vi "XMLExtractSheetData.vi"(8 "error in (no error)":errorcluster, 11 "SheetsXML":string[](array[string])=["<table:table table:name=\"Sheet1\" table:style-name=\"ta1\"><table:table-column table:style-name=\"co1\" table:number-columns-repeated=\"8\" table:default-cell-style-name=\"Default\"/><table:table-row table:style-name=\"ro1\" table:number-rows-repeated=\"3\"><table:table-cell table:number-columns-repeated=\"8\"/></table:table-row><table:table-row table:style-name=\"ro1\"><table:table-cell/><table:table-cell office:value-type=\"string\" calcext:value-type=\"string\"><text:p>b1</text:p></table:table-cell><table:table-cell office:value-type=\"string\" calcext:value-type=\"string\"><text:p>c1</text:p></table:table-cell><table:table-cell table:number-columns-repeated=\"5\"/></table:table-row><table:table-row table:style-name=\"ro1\"><table:table-cell/><table:table-cell office:value-type=\"string\" calcext:value-type=\"string\"><text:p>b2</text:p></table:table-cell><table:table-cell office:value-type=\"string\" calcext:value-type=\"string\"><text:p>c2</text:p></table:table-cell><table:table-cell table:number-columns-repeated=\"5\"/></table:table-row><table:table-row table:style-name=\"ro1\"><table:table-cell/><table:table-cell office:value-type=\"string\" calcext:value-type=\"string\"><text:p>b3</text:p></table:table-cell><table:table-cell office:value-type=\"string\" calcext:value-type=\"string\"><text:p>c3</text:p></table:table-cell><table:table-cell table:number-columns-repeated=\"5\"/></table:table-row><table:table-row table:style-name=\"ro1\"><table:table-cell/><table:table-cell office:value-type=\"string\" calcext:value-type=\"string\"><text:p>b4</text:p></table:table-cell><table:table-cell office:value-type=\"string\" calcext:value-type=\"string\"><text:p>c4</text:p></table:table-cell><table:table-cell table:number-columns-repeated=\"5\"/></table:table-row><table:table-row table:style-name=\"ro1\"><table:table-cell/><table:table-cell office:value-type=\"string\" calcext:value-type=\"string\"><text:p>b5</text:p></table:table-cell><table:table-cell office:value-type=\"string\" calcext:value-type=\"string\"><text:p>c5</text:p></table:table-cell><table:table-cell table:number-columns-repeated=\"5\"/></table:table-row><table:table-row table:style-name=\"ro1\"><table:table-cell/><table:table-cell office:value-type=\"string\" calcext:value-type=\"string\"><text:p>b6</text:p></table:table-cell><table:table-cell office:value-type=\"string\" calcext:value-type=\"string\"><text:p>c6</text:p></table:table-cell><table:table-cell table:number-columns-repeated=\"5\"/></table:table-row><table:table-row table:style-name=\"ro1\"><table:table-cell/><table:table-cell office:value-type=\"string\" calcext:value-type=\"string\"><text:p>b7</text:p></table:table-cell><table:table-cell office:value-type=\"string\" calcext:value-type=\"string\"><text:p>c7</text:p></table:table-cell><table:table-cell table:number-columns-repeated=\"5\"/></table:table-row><table:table-row table:style-name=\"ro1\"><table:table-cell/><table:table-cell office:value-type=\"string\" calcext:value-type=\"string\"><text:p>b8</text:p></table:table-cell><table:table-cell office:value-type=\"string\" calcext:value-type=\"string\"><text:p>c8</text:p></table:table-cell><table:table-cell table:number-columns-repeated=\"5\"/></table:table-row><table:table-row table:style-name=\"ro1\" table:number-rows-repeated=\"2\"><table:table-cell table:number-columns-repeated=\"8\"/></table:table-row><table:table-row table:style-name=\"ro1\"><table:table-cell table:number-columns-repeated=\"3\"/><table:table-cell office:value-type=\"string\" calcext:value-type=\"string\"><text:p>d1</text:p></table:table-cell><table:table-cell office:value-type=\"string\" calcext:value-type=\"string\"><text:p>e1</text:p></table:table-cell><table:table-cell table:number-columns-repeated=\"3\"/></table:table-row><table:table-row table:style-name=\"ro1\"><table:table-cell table:number-columns-repeated=\"3\"/><table:table-cell office:value-type=\"string\" calcext:value-type=\"string\"><text:p>d2</text:p></table:table-cell><table:table-cell office:value-type=\"string\" calcext:value-type=\"string\"><text:p>e2</text:p></table:table-cell><table:table-cell table:number-columns-repeated=\"3\"/></table:table-row><table:table-row table:style-name=\"ro1\"><table:table-cell table:number-columns-repeated=\"3\"/><table:table-cell office:value-type=\"string\" calcext:value-type=\"string\"><text:p>d3</text:p></table:table-cell><table:table-cell office:value-type=\"string\" calcext:value-type=\"string\"><text:p>e3</text:p></table:table-cell><table:table-cell table:number-columns-repeated=\"3\"/></table:table-row><table:table-row table:style-name=\"ro1\"><table:table-cell table:number-columns-repeated=\"3\"/><table:table-cell office:value-type=\"string\" calcext:value-type=\"string\"><text:p>d4</text:p></table:table-cell><table:table-cell office:value-type=\"string\" calcext:value-type=\"string\"><text:p>e4</text:p></table:table-cell><table:table-cell table:number-columns-repeated=\"3\"/></table:table-row><table:table-row table:style-name=\"ro1\"><table:table-cell table:number-columns-repeated=\"3\"/><table:table-cell office:value-type=\"string\" calcext:value-type=\"string\"><text:p>d5</text:p></table:table-cell><table:table-cell office:value-type=\"string\" calcext:value-type=\"string\"><text:p>e5</text:p></table:table-cell><table:table-cell table:number-columns-repeated=\"3\"/></table:table-row><table:table-row table:style-name=\"ro1\" table:number-rows-repeated=\"14\"><table:table-cell table:number-columns-repeated=\"8\"/></table:table-row><table:table-row table:style-name=\"ro1\"><table:table-cell table:number-columns-repeated=\"5\"/><table:table-cell office:value-type=\"string\" calcext:value-type=\"string\"><text:p>f1</text:p></table:table-cell><table:table-cell/><table:table-cell office:value-type=\"string\" calcext:value-type=\"string\"><text:p>h1</text:p></table:table-cell></table:table-row><table:table-row table:style-name=\"ro1\"><table:table-cell table:number-columns-repeated=\"5\"/><table:table-cell office:value-type=\"string\" calcext:value-type=\"string\"><text:p>f2</text:p></table:table-cell><table:table-cell/><table:table-cell office:value-type=\"string\" calcext:value-type=\"string\"><text:p>h2</text:p></table:table-cell></table:table-row><table:table-row table:style-name=\"ro1\"><table:table-cell table:number-columns-repeated=\"5\"/><table:table-cell office:value-type=\"string\" calcext:value-type=\"string\"><text:p>f3</text:p></table:table-cell><table:table-cell/><table:table-cell office:value-type=\"string\" calcext:value-type=\"string\"><text:p>h3</text:p></table:table-cell></table:table-row><table:table-row table:style-name=\"ro1\"><table:table-cell table:number-columns-repeated=\"5\"/><table:table-cell office:value-type=\"string\" calcext:value-type=\"string\"><text:p>f4</text:p></table:table-cell><table:table-cell/><table:table-cell office:value-type=\"string\" calcext:value-type=\"string\"><text:p>h4</text:p></table:table-cell></table:table-row><table:table-row table:style-name=\"ro1\"><table:table-cell table:number-columns-repeated=\"5\"/><table:table-cell office:value-type=\"string\" calcext:value-type=\"string\"><text:p>f5</text:p></table:table-cell><table:table-cell/><table:table-cell office:value-type=\"string\" calcext:value-type=\"string\"><text:p>h5</text:p></table:table-cell></table:table-row><table:table-row table:style-name=\"ro1\"><table:table-cell table:number-columns-repeated=\"5\"/><table:table-cell office:value-type=\"string\" calcext:value-type=\"string\"><text:p>f6</text:p></table:table-cell><table:table-cell/><table:table-cell office:value-type=\"string\" calcext:value-type=\"string\"><text:p>h6</text:p></table:table-cell></table:table-row><table:table-row table:style-name=\"ro1\"><table:table-cell table:number-columns-repeated=\"5\"/><table:table-cell office:value-type=\"string\" calcext:value-type=\"string\"><text:p>f7</text:p></table:table-cell><table:table-cell/><table:table-cell office:value-type=\"string\" calcext:value-type=\"string\"><text:p>h7</text:p></table:table-cell></table:table-row></table:table>"]) -> (0 "error out":errorcluster, 2 "SpreadsheetData":T1[](array[typedef]), 3 "Table HeaderInfo":string[](array[string]))   [LabVIEW 2014]
uses:
  Spreadsheets.ctl
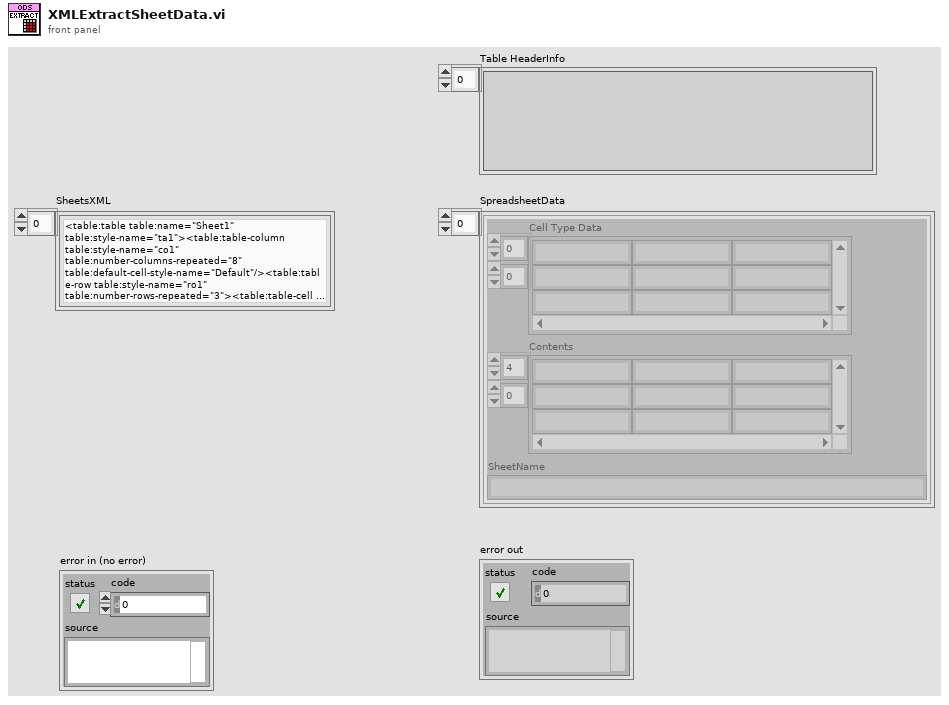
[diagram p1: front panel]
types:
  T1 = typedef "Spreadsheets.ctl" = cluster{"Cell Type Data":string[][], "Contents":string[][], "SheetName":string}
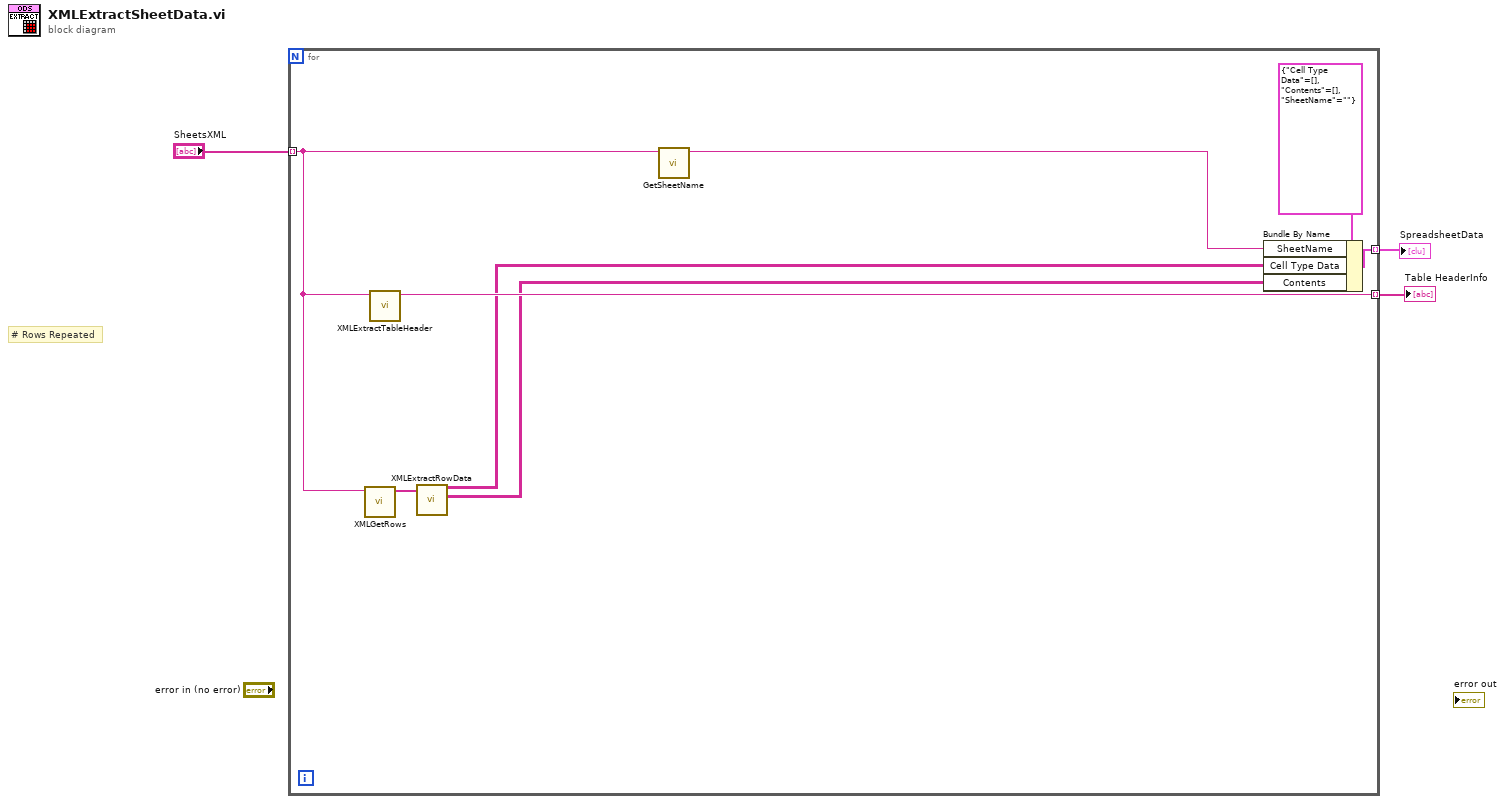
[diagram p0: block diagram]
diagram:
  # "# Rows Repeated"
  n1 = for {
    tunnel: "SheetsXML" -> [w7] mode=indexing
    tunnel: [w10] -> w2 mode=indexing
    tunnel: [w8] -> w1 mode=indexing
    n2 = call "XMLGetRows.vi"("XML"=w7) -> ("Rows"=w6:string[])  [unwired: 10 in]
    n3 = call "XMLExtractTableHeader.vi"("XMLIn"=w7) -> ("TableHeaderInfo"=w8:string)  [unwired: 10 in]
    n4 = call "XMLExtractRowData.vi"("Rows"=w6) -> ("Contents"=w4:string[][], "Cell Type Data"=w5:string[][])  [unwired: 9 in]
    n5 = call "GetSheetName.vi"("String"=w7) -> ("whole match"=w9:string)  [unwired: 10 in]
    n6 = Bundle By Name(cluster=T1 {"Cell Type Data"=[], "Contents"=[], "SheetName"=""} ("Sheet"), "SheetName"=w9, "Cell Type Data"=w5, "Contents"=w4) -> (w10:T1)
  }
  "SpreadsheetData" <- w2
  "Table HeaderInfo" <- w1
